vi "get_status.vi"(11 "REST Client in":refnum<class "REST Client.lvclass">) -> (0 "error out":errorcluster, 1 "car_status":T1, 2 "Response body":string, 3 "REST Client out":refnum<class "REST Client.lvclass">)   [LabVIEW 2024]
uses:
  <vilib>/addons/_JKI.lib/REST Client/classes/REST Client/REST Client.lvclass
  typeDef/car_status.ctl
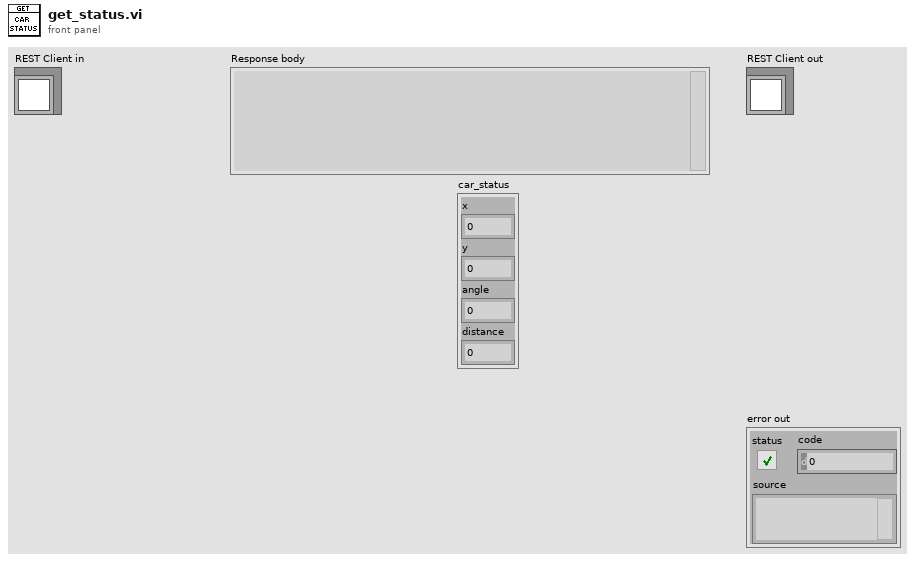
[diagram p1: front panel]
types:
  T1 = typedef "car_status.ctl" = cluster{"x":dbl, "y":dbl, "angle":dbl, "distance":dbl}
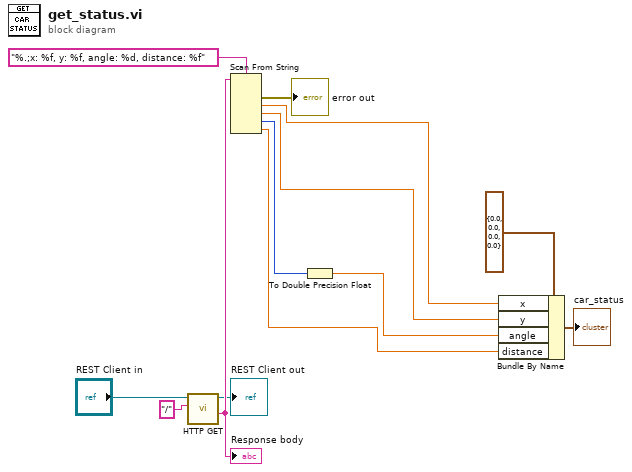
[diagram p0: block diagram]
diagram:
  n1 = call-dynamic "HTTP GET.vi"("Path"="/", "REST Client in"="REST Client in") -> ("Response body"=w9:string, "REST Client out"=→"REST Client out":refnum<class "REST Client.lvclass">)  [unwired: 4 in, 4 out]
  "Response body" <- w9
  n2 = Scan From String(format string="%.;x: %f, y: %f, angle: %d, distance: %f", input string=w9) -> (error out=→"error out":errorcluster, output 1=w5:dbl, output 2=w4:dbl, output 3=w12:i32, output 4=w2:dbl)  [unwired: 6 in, 2 out]
  n3 = To Double Precision Float(number=w12) -> (double precision float=w3:dbl)
  n4 = Bundle By Name(cluster=T1 {"x"=0.0, "y"=0.0, "angle"=0.0, "distance"=0.0}, "x"=w5, "y"=w4, "angle"=w3, "distance"=w2) -> (→"car_status":T1)
